vi "MoveCommands (SubVI).vi"() -> (3 "MoveCommands":T1)   [LabVIEW 2018]
uses:
  TypeDefs/MoveCommands.ctl
panel:
  # "0 - 48 ASCII"
  # "1 - 49 ASCII"
  # "2 - 50 ASCII"
  # "3 - 51 ASCII"
  # "4 - 52 ASCII"
  # "5 - 53 ASCII"
  # "6 - 54 ASCII"
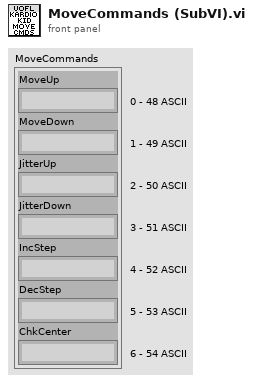
[diagram p1: front panel]
types:
  T1 = typedef "MoveCommands.ctl" = cluster{"MoveUp":string, "MoveDown":string, "JitterUp":string, "JitterDown":string, "IncStep":string, "DecStep":string, "ChkCenter":string}
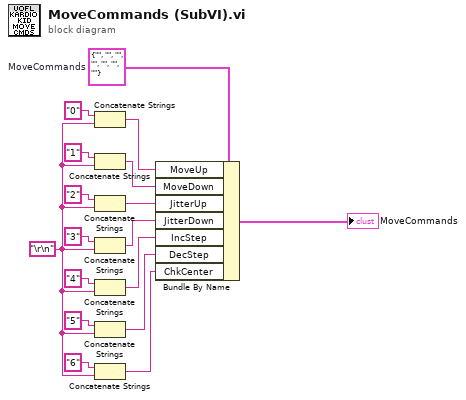
[diagram p0: block diagram]
diagram:
  w3 = T1 {"MoveUp"="", "MoveDown"="", "JitterUp"="", "JitterDown"="", "IncStep"="", "DecStep"="", "ChkCenter"=""}  # MoveCommands
  w16 = "\r\n"
  n1 = Concatenate Strings("0", w16) -> (w2:string)
  n2 = Concatenate Strings("1", w16) -> (w7:string)
  n3 = Concatenate Strings("2", w16) -> (w8:string)
  n4 = Concatenate Strings("3", w16) -> (w9:string)
  n5 = Concatenate Strings("4", w16) -> (w12:string)
  n6 = Concatenate Strings("5", w16) -> (w13:string)
  n7 = Concatenate Strings("6", w16) -> (w15:string)
  n8 = Bundle By Name(cluster=w3, "MoveUp"=w2, "MoveDown"=w7, "JitterUp"=w8, "JitterDown"=w9, "IncStep"=w12, "DecStep"=w13, "ChkCenter"=w15) -> (→"MoveCommands":T1)
